vi "Finalize To Settings.vi"(8 "error in (no error)":errorcluster, 11 "User Interface in":refnum<class "User Interface.lvclass">) -> (0 "error out":errorcluster, 2 "settings":cluster{"key":string, "value":string}[](array[cluster]), 3 "User Interface out":refnum<class "User Interface.lvclass">)   [LabVIEW 2019, in "DSF Core.lvlib" / "User Interface.lvclass"]
uses:
  User Interface.lvclass
  User Interface.lvclass/User Interface.ctl
  Configuration/Configuration.lvclass
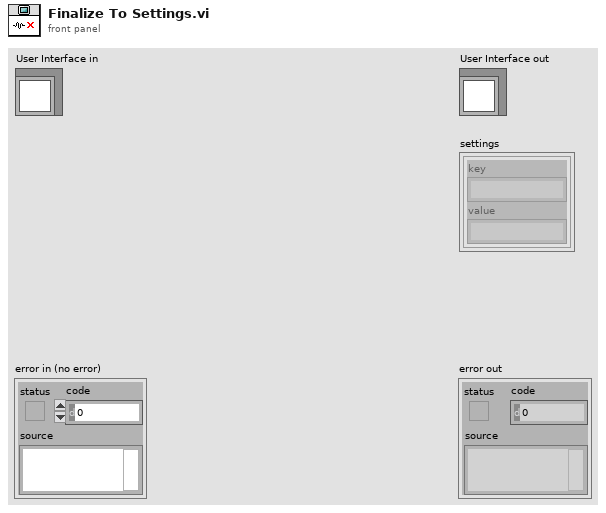
[diagram p1: front panel]
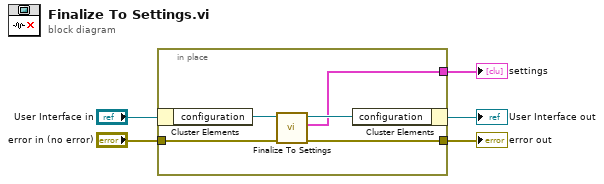
[diagram p0: block diagram]
diagram:
  n1 = in-place {
    in-place-border: "error in (no error)" -> [w9]
    in-place-border: [w7] -> w2
    in-place-border: [w6] -> w1
    n2 = in-place-cluster #1("User Interface in") -> ("configuration"=w10:refnum<class "Configuration.lvclass">)
    n3 = call-dynamic "Finalize To Settings.vi"("error in (no error)"=w9, "Configuration in"=w10) -> ("error out"=w7:errorcluster, "settings"=w6:cluster{"key":string, "value":string}[], "Configuration out"=w8:refnum<class "Configuration.lvclass">)  [unwired: 7 in]
    n4 = in-place-cluster #1("configuration"=w8) -> (→"User Interface out":refnum<class "User Interface.lvclass">)
  }
  "error out" <- w2
  "settings" <- w1
